vi "Read Product Sub Panel.vi"(8 "error in (no error)":errorcluster, 11 "Prooduct Actor in":refnum<class "Prooduct Actor.lvclass">) -> (0 "error out":errorcluster, 2 "Product Sub Panel":refnum<vi>, 3 "Prooduct Actor out":refnum<class "Prooduct Actor.lvclass">)   [LabVIEW 2020, in "Prooduct Actor.lvlib" / "Prooduct Actor.lvclass"]
uses:
  Prooduct Actor.lvclass
  Prooduct Actor.lvclass/Prooduct Actor.ctl
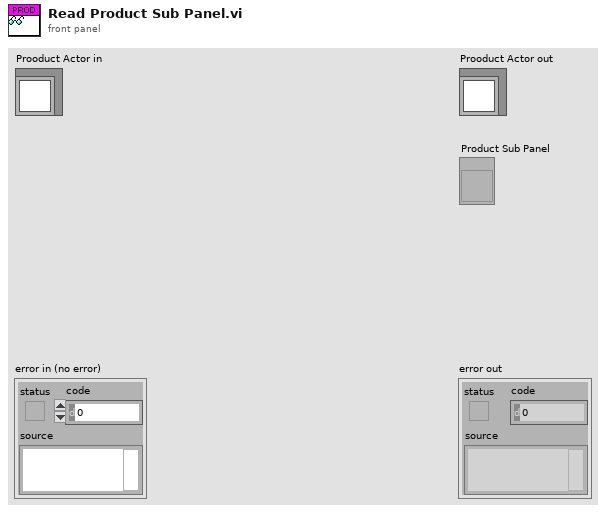
[diagram p1: front panel]
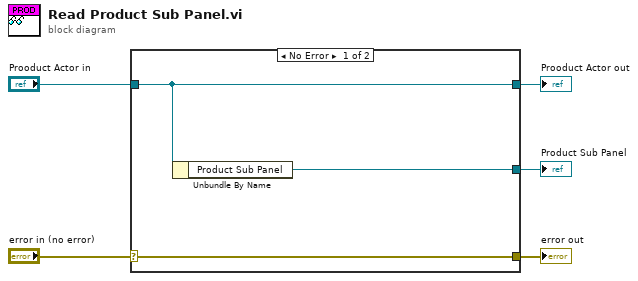
[diagram p0: block diagram]
diagram:
  n1 = case shown="No Error" "error in (no error)" {
    selector: "error in (no error)" -> [w8 w9]
    tunnel: [w8 w9] -> w4
    tunnel: [w7 w10] -> w2
    tunnel: "Prooduct Actor in" -> [w7 w10]
    tunnel: [w6 _] -> w1
    frame No Error {
      n2 = Unbundle By Name(w7) -> ("Product Sub Panel"=w6:refnum<vi>)
    }
    frame Error {
    }
  }
  "error out" <- w4
  "Prooduct Actor out" <- w2
  "Product Sub Panel" <- w1
